vi "Table Function - Copy to Ext-Clipboard.vi"(8 "error in":errorcluster, 9 "Selection Size":T1, 10 "Selection Start":T1, 11 "Text Table In":string[][](array[string])) -> (0 "error out":errorcluster, 1 "Cut Section to Clipboard":string[][](array[string]), 3 "Text Table Out":string[][](array[string]))   [LabVIEW 2018]
uses:
  <vilib>/Utility/miscctls.llb/LVRowAndColumnTypeDef.ctl
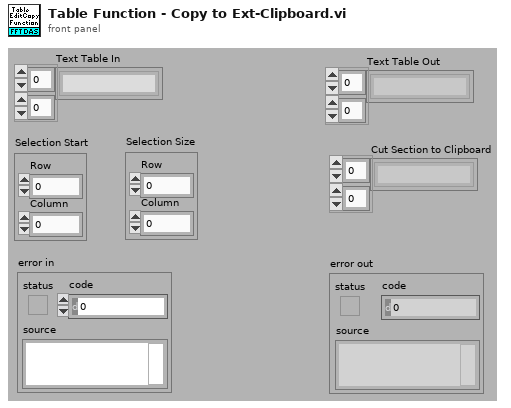
[diagram p1: front panel]
types:
  T1 = typedef "LVRowAndColumnTypeDef.ctl" = cluster{"Row":i32, "Column":i32}
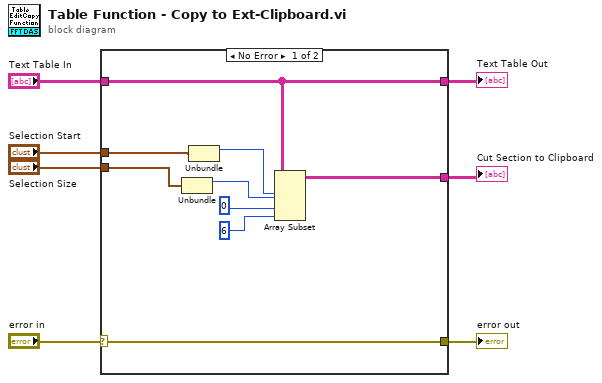
[diagram p0: block diagram]
diagram:
  n1 = case shown="No Error" "error in" {
    selector: "error in" -> [w16 w17]
    tunnel: "Selection Size" -> [w10 _]
    tunnel: "Selection Start" -> [w11 _]
    tunnel: [w9 w18] -> w5
    tunnel: "Text Table In" -> [w9 w18]
    tunnel: [w8 _] -> w3
    tunnel: [w16 w17] -> w1
    frame No Error {
      n2 = Unbundle(w10) -> ("Row"=w13:i32)  [unwired: 1 out]
      n3 = Unbundle(w11) -> ("Row"=w12:i32)  [unwired: 1 out]
      n4 = Array Subset(array=w9, index (row)=w12, length (row)=w13, index (col)=0, length (col)=6) -> (w8:string[][])
    }
    frame Error {
    }
  }
  "Text Table Out" <- w5
  "Cut Section to Clipboard" <- w3
  "error out" <- w1
